vi "TestEvaluator_Init.vi"(0 "object in":refnum<class "TestEvaluator.lvclass">, 5 "error in (no error)":errorcluster) -> (14 "object out":refnum<class "TestEvaluator.lvclass">, 19 "error out":errorcluster)   [LabVIEW 2023, in "TestEvaluator.lvclass"]
uses:
  TestEvaluator.lvclass
  C:/Users/ebert/Documents/codes/SSL/repo/SSL_AI/NewSTP/Evaluators/Evaluator_class/Evaluator.lvclass
  Criteria/ReceptionAngle_class/ReceptionAngle.lvclass
  C:/Users/ebert/Documents/codes/SSL/repo/SSL_AI/NewSTP/Criteria/Criterion_class/Criterion.lvclass
  Criteria/OpenAngleToGoal_class/OpenAngleToGoal.lvclass
  Criteria/OutOfGoalieArea_class/OutOfGoalieArea.lvclass
  Evaluator_class/Evaluator.lvclass
  Criteria/Criterion_class/Criterion.lvclass
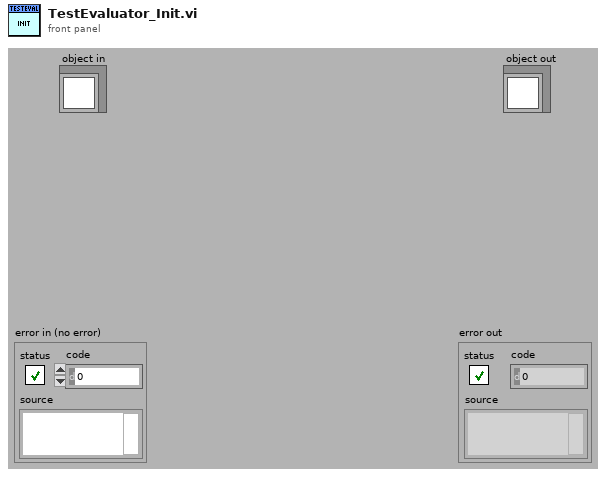
[diagram p1: front panel]
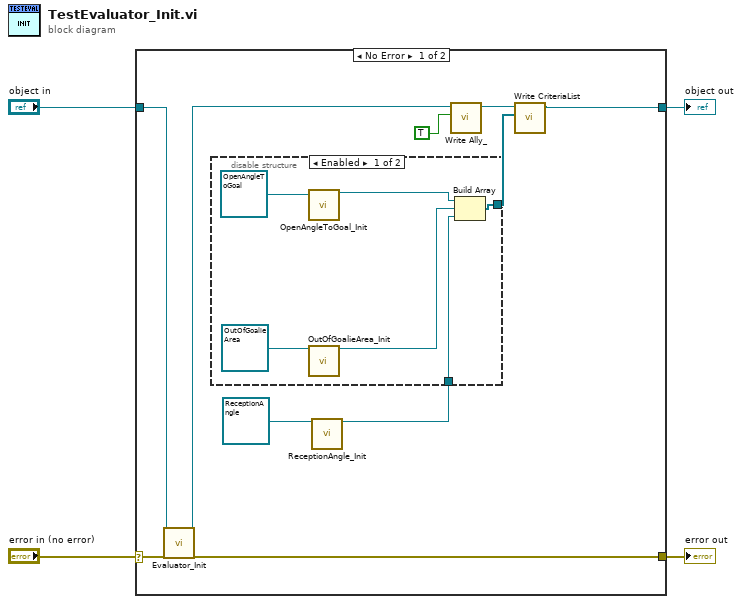
[diagram p0: block diagram]
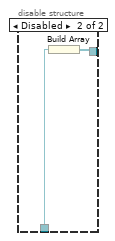
[diagram p2: hidden frame]
diagram:
  n1 = case shown="No Error" "error in (no error)" {
    selector: "error in (no error)" -> [w14 w23]
    tunnel: [w8 w24] -> w4
    tunnel: "object in" -> [w12 w24]
    tunnel: [w13 w23] -> w1
    frame No Error {
      n2 = call "Evaluator_Init.vi"("object in"=w12, "error in (no error)"=w14) -> ("object out"=w11:refnum<class "TestEvaluator.lvclass">, "error out"=w13:errorcluster)  [unwired: 16 in]
      n3 = call "ReceptionAngle_Init.vi"("object in"=refnum<class "ReceptionAngle.lvclass"> refnum ("ReceptionAngle")) -> ("object out"=w6:refnum<class "ReceptionAngle.lvclass">)  [unwired: 17 in, 1 out]
      n4 = disable-structure shown="Enabled" {
        disable-tunnel: w6 -> [w17 w22]
        disable-tunnel: [w16 w21] -> w5
        frame Enabled {
          n5 = call "OpenAngleToGoal_Init.vi"("object in"=refnum<class "OpenAngleToGoal.lvclass"> refnum ("OpenAngleToGoal")) -> ("object out"=w15:refnum<class "OpenAngleToGoal.lvclass">)  [unwired: 17 in, 1 out]
          n6 = call "OutOfGoalieArea_Init.vi"("object in"=refnum<class "OutOfGoalieArea.lvclass"> refnum ("OutOfGoalieArea")) -> ("object out"=w18:refnum<class "OutOfGoalieArea.lvclass">)  [unwired: 17 in, 1 out]
          n7 = Build Array(w15, w18, w17) -> (w16:refnum<class "Criterion.lvclass">[])
        }
        frame Disabled {
          n8 = Build Array(w22) -> (w21:refnum<class "ReceptionAngle.lvclass">[])
        }
      }
      n9 = call-dynamic "Write Ally_.vi"("Ally?"=TRUE, "Evaluator in"=w11) -> ("Evaluator out"=w10:refnum<class "TestEvaluator.lvclass">)  [unwired: 8 in, 1 out]
      n10 = call-dynamic "Write CriteriaList.vi"("CriteriaList"=w5, "Evaluator in"=w10) -> ("Evaluator out"=w8:refnum<class "TestEvaluator.lvclass">)  [unwired: 8 in, 1 out]
    }
    frame Error {
    }
  }
  "object out" <- w4
  "error out" <- w1
